vi "TestSubpanel.vi"(11 "Error In":errorcluster) -> (15 "Error Out":errorcluster)   [LabVIEW 2016, in "SubpanelTests.lvlib"]
doc: "Test boolean and numeric controls within subpanel"
uses:
  SubpanelTests.lvlib
  APIs/Stimulus/VI/MakeVIFrontMost.vi
  APIs/Stimulus/ControlValue/ValueSignalByPathString.vi
  APIs/Stimulus/ControlValue/ValueSignalLatchBooleanString.vi
  APIs/Stimulus/VI/CloseVI.vi
  <vilib>/addons/_JKI Toolkits/Caraya/classes/Test/Test.lvclass
  Drona.lvlib
  APIs/Stimulus/ControlValue/ControlValue.lvlib
  APIs/Stimulus/VI/VI.lvlib
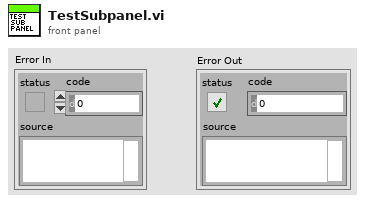
[diagram p1: front panel]
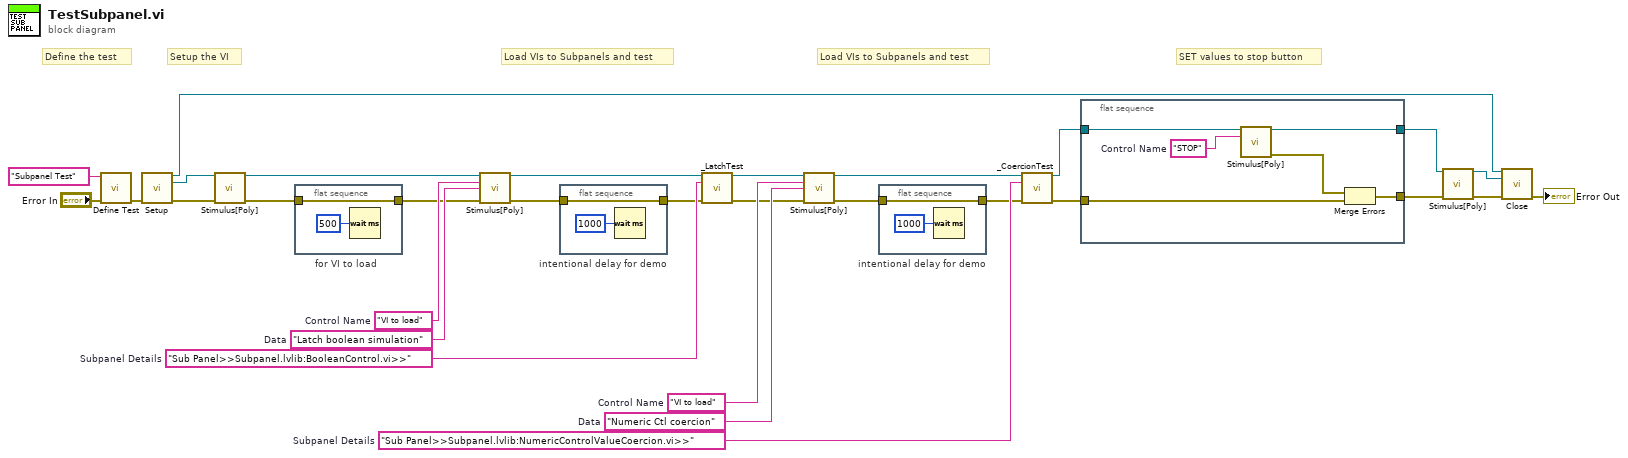
[diagram p0: block diagram]
diagram:
  w22 = "Sub Panel>>Subpanel.lvlib:BooleanControl.vi>>"  # Subpanel Details
  w25 = "Latch boolean simulation"  # Data
  w24 = "VI to load"  # Control Name
  w26 = "Sub Panel>>Subpanel.lvlib:NumericControlValueCoercion.vi>>"  # Subpanel Details
  w28 = "Numeric Ctl coercion"  # Data
  w29 = "VI to load"  # Control Name
  # "Load VIs to Subpanels and test"
  # "Load VIs to Subpanels and test"
  # "SET values to stop button"
  # "Setup the VI"
  # "Define the test"
  n1 = call <vilib>:"Define Test.vi"("error in (no error)"="Error In", "Label (VI Title)"="Subpanel Test") -> ("error out"=w12:errorcluster)  [unwired: 9 in]
  n2 = call "Setup.vi"("error in"=w12) -> ("Application Ref"=w7:refnum<vi>, "VI Reference Out"=w9:refnum<vi>, "error out"=w11:errorcluster)  [unwired: 12 in]
  n3 = call-poly "Stimulus[Poly].vi"("VI Reference In"=w9, "error in"=w11) -> ("VI Reference Out"=w8:refnum<vi>, "error out"=w10:errorcluster)  [unwired: 12 in]
  n4 = flat-sequence "for VI to load" {
    tunnel: w10 -> [w31]
    tunnel: [w31] -> w13
    frame #0 {
      n5 = Wait (ms)(milliseconds to wait=u32 500) -> ()  [unwired: 1 out]
    }
  }
  n6 = call-poly "Stimulus[Poly].vi"("VI Reference In"=w8, "Control Path"=w24, "Value (Signaling)"=w25, "error in"=w13) -> ("VI Reference Out"=w23:refnum<vi>, "error out"=w17:errorcluster)  [unwired: 10 in]
  n7 = flat-sequence "intentional delay for demo" {
    tunnel: w17 -> [w33]
    tunnel: [w33] -> w16
    frame #0 {
      n8 = Wait (ms)(milliseconds to wait=u32 1000) -> ()  [unwired: 1 out]
    }
  }
  n9 = call "_LatchTest.vi"("VI Reference In"=w23, "Subpanel Details"=w22, "Error In"=w16) -> ("VI Reference Out"=w21:refnum<vi>, "Error Out"=w20:errorcluster)  [unwired: 11 in]
  n10 = call-poly "Stimulus[Poly].vi"("VI Reference In"=w21, "Control Path"=w29, "Value (Signaling)"=w28, "error in"=w20) -> ("VI Reference Out"=w27:refnum<vi>, "error out"=w15:errorcluster)  [unwired: 10 in]
  n11 = flat-sequence "intentional delay for demo" {
    tunnel: w15 -> [w35]
    tunnel: [w35] -> w14
    frame #0 {
      n12 = Wait (ms)(milliseconds to wait=u32 1000) -> ()  [unwired: 1 out]
    }
  }
  n13 = call "_CoercionTest.vi"("VI Reference In"=w27, "Subpanel Details"=w26, "Error In"=w14) -> ("VI Reference Out"=w18:refnum<vi>, "Error Out"=w19:errorcluster)  [unwired: 11 in]
  n14 = flat-sequence {
    tunnel: [w41] -> w4
    tunnel: [w42] -> w3
    tunnel: w19 -> [w38]
    tunnel: w18 -> [w37]
    frame #0 {
      w39 = "STOP"  # Control Name
      n15 = call-poly "Stimulus[Poly].vi"("VI Reference In"=w37, "Control Path"=w39) -> ("VI Reference Out"=w42:refnum<vi>, "error out"=w40:errorcluster)  [unwired: 12 in]
      n16 = Merge Errors(w40, w38) -> (w41:errorcluster)
    }
  }
  n17 = call-poly "Stimulus[Poly].vi"("VI Reference In"=w3, "error in"=w4) -> ("VI Reference Out"=w2:refnum<vi>, "error out"=w1:errorcluster)  [unwired: 12 in]
  n18 = call "Close.vi"("Application Ref"=w7, "VI Reference"=w2, "error in"=w1) -> ("error out"=→"Error Out":errorcluster)  [unwired: 12 in]
